vi "DPT Config Write.vi"(0 "Config File Path":path=path "C:/work/flowconfig.ini", 11 "error in (no error)":errorcluster) -> (15 "error out":errorcluster)   [LabVIEW 2009]
uses:
  <vilib>/Utility/config.llb/Write Key (String).vi
  Global Test Variables DPT.vi
  <vilib>/Utility/config.llb/NI_LVConfig.lvlib
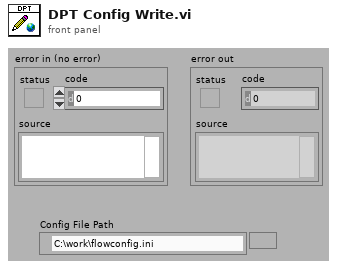
[diagram p1: front panel]
types:
  T1 = typedef "NI_LVConfig.lvlib/Config Data RefNum.ctl" = refnum<k1>
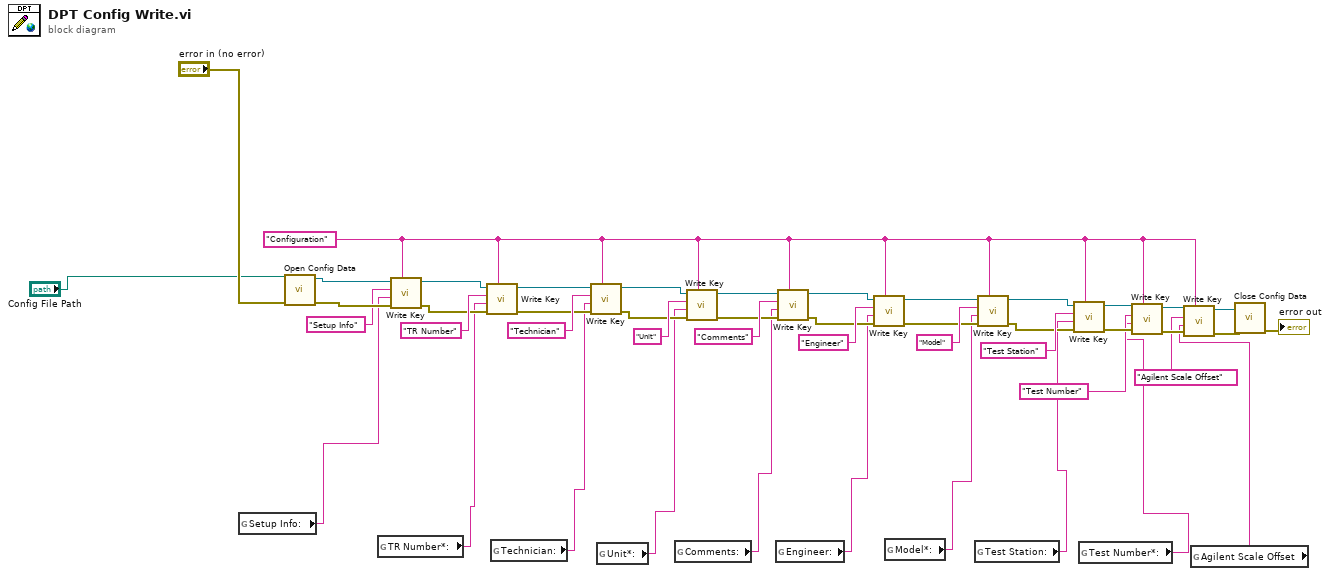
[diagram p0: block diagram]
diagram:
  w3 = "Configuration" ("key")
  n1 = global read "Global Test Variables DPT.vi" "Setup Info:"() -> (w16:string)
  n2 = call <vilib>:"Open Config Data.vi"("error in (no error)"="error in (no error)", "configuration file path"="Config File Path") -> ("error out"=w42:errorcluster, "refnum"=w43:T1)  [unwired: 7 in, 1 out]
  n3 = global read "Global Test Variables DPT.vi" "TR Number*:"() -> (w15:string)
  n4 = call-poly <vilib>:"Write Key.vi"("section"=w3, "error in (no error)"=w42, "value"=w16, "key"="Setup Info", "refnum"=w43) -> ("error out"=w39:errorcluster, "refnum out"=w34:T1)  [unwired: 4 in, 1 out]
  n5 = call-poly <vilib>:"Write Key.vi"("section"=w3, "error in (no error)"=w39, "value"=w15, "key"="TR Number", "refnum"=w34) -> ("error out"=w35:errorcluster, "refnum out"=w33:T1)  [unwired: 4 in, 1 out]
  n6 = global read "Global Test Variables DPT.vi" "Technician:"() -> (w14:string)
  n7 = call-poly <vilib>:"Write Key.vi"("section"=w3, "error in (no error)"=w35, "value"=w14, "key"="Technician", "refnum"=w33) -> ("error out"=w36:errorcluster, "refnum out"=w32:T1)  [unwired: 4 in, 1 out]
  n8 = global read "Global Test Variables DPT.vi" "Unit*:"() -> (w13:string)
  n9 = global read "Global Test Variables DPT.vi" "Comments:"() -> (w12:string)
  n10 = call-poly <vilib>:"Write Key.vi"("section"=w3, "error in (no error)"=w36, "value"=w13, "key"="Unit", "refnum"=w32) -> ("error out"=w20:errorcluster, "refnum out"=w21:T1)  [unwired: 4 in, 1 out]
  n11 = global read "Global Test Variables DPT.vi" "Engineer:"() -> (w11:string)
  n12 = call-poly <vilib>:"Write Key.vi"("section"=w3, "error in (no error)"=w20, "value"=w12, "key"="Comments", "refnum"=w21) -> ("error out"=w29:errorcluster, "refnum out"=w24:T1)  [unwired: 4 in, 1 out]
  n13 = call-poly <vilib>:"Write Key.vi"("section"=w3, "error in (no error)"=w29, "value"=w11, "key"="Engineer", "refnum"=w24) -> ("error out"=w25:errorcluster, "refnum out"=w23:T1)  [unwired: 4 in, 1 out]
  n14 = global read "Global Test Variables DPT.vi" "Model*:"() -> (w10:string)
  n15 = global read "Global Test Variables DPT.vi" "Test Station:"() -> (w9:string)
  n16 = call-poly <vilib>:"Write Key.vi"("section"=w3, "error in (no error)"=w25, "value"=w10, "key"="Model", "refnum"=w23) -> ("error out"=w26:errorcluster, "refnum out"=w22:T1)  [unwired: 4 in, 1 out]
  n17 = call-poly <vilib>:"Write Key.vi"("section"=w3, "error in (no error)"=w26, "value"=w9, "key"="Test Station", "refnum"=w22) -> ("error out"=w18:errorcluster, "refnum out"=w19:T1)  [unwired: 4 in, 1 out]
  n18 = global read "Global Test Variables DPT.vi" "Test Number*:"() -> (w8:string)
  n19 = call-poly <vilib>:"Write Key.vi"("section"=w3, "error in (no error)"=w18, "value"=w8, "key"="Test Number", "refnum"=w19) -> ("error out"=w6:errorcluster, "refnum out"=w7:T1)  [unwired: 4 in, 1 out]
  n20 = global read "Global Test Variables DPT.vi" "Agilent Scale Offset"() -> (w2:string)
  n21 = call-poly <vilib>:"Write Key.vi"("section"=w3, "error in (no error)"=w6, "value"=w2, "key"="Agilent Scale Offset", "refnum"=w7) -> ("error out"=w5:errorcluster, "refnum out"=w4:T1)  [unwired: 4 in, 1 out]
  n22 = call <vilib>:"Close Config Data.vi"("error in (no error)"=w5, "refnum"=w4) -> ("error out"=→"error out":errorcluster)  [unwired: 8 in, 1 out]
